vi "Recieve IP.vi"(11 "Stop":bool) -> (3 "String":string)   [LabVIEW 2016]
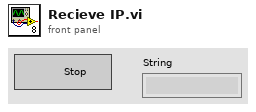
[diagram p1: front panel]
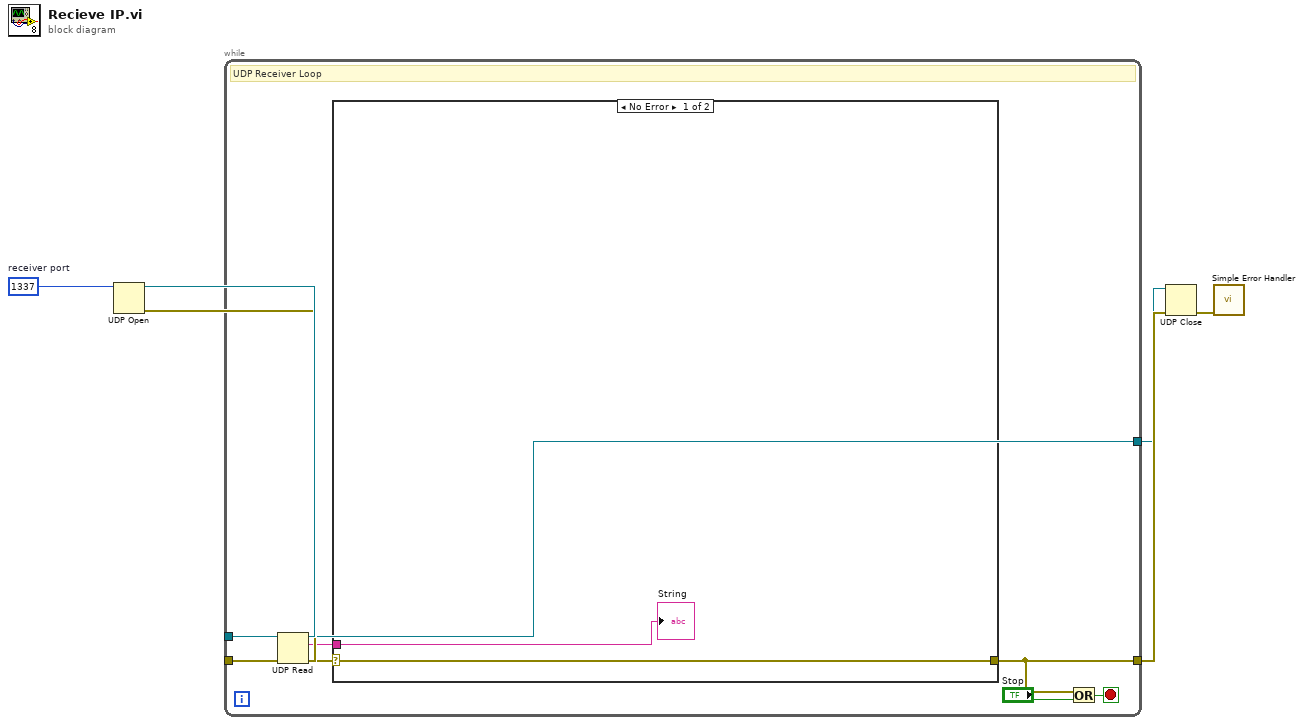
[diagram p0: block diagram]
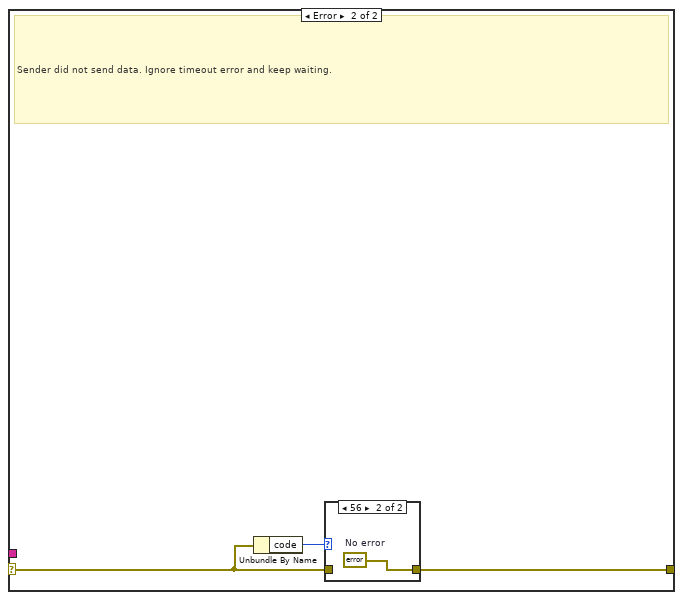
[diagram p2: hidden frame]
diagram:
  w6 = u16 1337  # receiver port
  n1 = UDP Open(11:w6) -> (port=w5:refnum<k16>, 0:w4:errorcluster)  [unwired: 4 in, 1 out]
  n2 = while {
    tunnel: w5 -> [w14]
    tunnel: [w7] -> w1
    tunnel: w4 -> [w11]
    tunnel: [w8] -> w3
    stop <- w12 stop-if-true
    # "UDP Receiver Loop"
    n3 = UDP Read(connection ID=w14, 8:w11) -> (data out=w10:string, error out=w9:errorcluster, 3:w7:refnum<k16>)  [unwired: 1 in, 3 out]
    n4 = case shown="No Error" w9 {
      selector: w9 -> [w16 w18]
      tunnel: w10 -> [w15 _]
      tunnel: [w16 w17] -> w8
      frame No Error {
        "String" <- w15
      }
      frame Error {
        # "Sender did not send data. Ignore timeout error and keep waiting."
        n5 = Unbundle By Name(w18) -> ("code"=w19:i32)
        n6 = case shown="56" w19 {
          tunnel: w18 -> [w20 _]
          tunnel: [w20 w21] -> w17
          frame Default {
          }
          frame 56 {
            w21 = errorcluster {"status"=FALSE, "code"=0, "source"=""}  # No error
          }
        }
      }
    }
    n7 = Or(x=w8, y="Stop") -> (x .or. y?=w12:bool)
  }
  n8 = UDP Close(connection ID=w1, 8:w3) -> (error out=w2:errorcluster)  [unwired: 1 out]
  n9 = call <vilib>:"Simple Error Handler.vi"("error in (no error)"=w2) -> ()  [unwired: 1 in, 8 out]
